vi "move.vi"(0 "value( disatance or angle)":dbl=1000.0 format="%#_13g", 1 "Speed precent":dbl(slide)=1.0 scale=0.0..1.0, 2 "mode":string="S") -> ()   [LabVIEW 2017]
uses:
  <vilib>/myRIO/Express VI/Onboard IO/PWM/PWM Express VI.xnode
  <vilib>/myRIO/Instrument Drivers/Onboard IO/PWM/vis/Set Duty Cycle and Frequency.vi
  <vilib>/myRIO/Instrument Drivers/Onboard IO/PWM/PWM.lvlib
  <vilib>/myRIO/Instrument Drivers/Onboard IO/PWM/typedefs/PWM Configuration.ctl
  <vilib>/myRIO/Common/Instrument Driver Framework/myRIO v1.0/PWM/typedefs/PWM Channels Enum.ctl
  <vilib>/myRIO/Common/Instrument Driver Framework/Utilities/typedefs/Generic FPGA Reference.ctl
  <vilib>/myRIO/Common/Instrument Driver Framework/Utilities/typedefs/myRIO v1.0 Reference.ctl
  <vilib>/myRIO/Common/Instrument Driver Framework/Utilities/typedefs/Hardware Version Enum.ctl
  <vilib>/myRIO/Common/Instrument Driver Framework/Utilities/typedefs/myRIO Generic Hardware Reference.ctl
  <vilib>/myRIO/Instrument Drivers/Onboard IO/PWM/typedefs/PWM Reference.ctl
  <vilib>/myRIO/Instrument Drivers/Onboard IO/PWM/vis/myRIO PWM Open.xnode
  <vilib>/myRIO/Common/Instrument Driver Framework/Utilities/vis/Is FPGA Ref Available.vi
  <vilib>/myRIO/Common/Instrument Driver Framework/myRIO v1.0/PWM/vis/myRIO v1.1 Open PWM.vi
  <vilib>/userdefined/High Color/nirio_resource_hc.ctl
  <vilib>/myRIO/Express VI/Onboard IO/DO/DO Express VI.xnode
  <vilib>/myRIO/Instrument Drivers/Onboard IO/DIO/vis/Write.vi
  <vilib>/myRIO/Instrument Drivers/Onboard IO/DIO/DIO.lvlib
  <vilib>/myRIO/Common/Instrument Driver Framework/myRIO v1.0/DIO/typedefs/DIO Channels Enum.ctl
  <vilib>/myRIO/Common/Instrument Driver Framework/myRIO v1.0/DIO/typedefs/DIO Channels List.ctl
  <vilib>/myRIO/Instrument Drivers/Onboard IO/DIO/typedefs/DIO Reference.ctl
  <vilib>/myRIO/Instrument Drivers/Onboard IO/DIO/vis/myRIO DIO Open.xnode
  <vilib>/myRIO/Common/Instrument Driver Framework/myRIO v1.0/DIO/vis/myRIO v1.1 Open DIO.vi
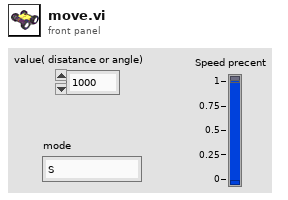
[diagram p1: front panel]
types:
  T1 = typedef "DIO.lvlib/DIO Reference.ctl" = cluster{"myRIO Reference":T2, "DIO Channels List":T6}
  T2 = typedef "myRIO Generic Hardware Reference.ctl" = cluster{"myRIO Model":T3, "myRIO Hardware Reference":T4}
  T3 = typedef "Hardware Version Enum.ctl" = enum16{"Unknown", "myRIO-1900", "myRIO-1950", "roboRIO", "NI ELVIS RIO CM"}
  T4 = typedef "myRIO v1.0 Reference.ctl" = cluster{"Generic FPGA Reference":T5, "Allow multiple opens":bool}
  T5 = typedef "Generic FPGA Reference.ctl" = refnum<k20>
  T6 = typedef "DIO Channels List.ctl" = T7[]
  T7 = typedef "DIO Channels Enum.ctl" = enum16{"Not Connected", "C/DIO0", "C/DIO1", "C/DIO2", "C/DIO3", "C/DIO4", "C/DIO5", "C/DIO6", "C/DIO7", "A/DIO0", "A/DIO1", "A/DIO2", "A/DIO3", "A/DIO4", "A/DIO5", "A/DIO6", "A/DIO7", "A/DIO8", "A/DIO9", "A/DIO10", "A/DIO11", "A/DIO12", "A/DIO13", "A/DIO14", "A/DIO15", "B/DIO0", "B/DIO1", "B/DIO2", "B/DIO3", "B/DIO4", "B/DIO5", "B/DIO6", "B/DIO7", "B/DIO8", "B/DIO9", "B/DIO10", "B/DIO11", "B/DIO12", "B/DIO13", "B/DIO14", "B/DIO15", "LED0", "LED1", "LED2", "LED3", "Button0", "DIO/DIO0", "DIO/DIO1", "DIO/DIO2", "DIO/DIO3", "DIO/DIO4", "DIO/DIO5", "DIO/DIO6", "DIO/DIO7", "DIO/DIO8", "DIO/DIO9", "SPI/CS0", "SPI/CS1", "SPI/CS2", "SPI/CS3", "LED RADIO (Green)", "LED RADIO (Red)", "LED COMM (Green)", "LED COMM (Red)", "LED MODE (Green)", "LED MODE (Red)"}
  T8 = typedef "nirio_resource_hc.ctl" = tag
  T9 = typedef "PWM.lvlib/PWM Reference.ctl" = cluster{"myRIO Reference":T2, "PWM Channels Enum":T10, "PWM Configuration":T11}
  T10 = typedef "PWM Channels Enum.ctl" = enum16{"Not Connected", "C/PWM0", "C/PWM1", "A/PWM0", "A/PWM1", "A/PWM2", "B/PWM0", "B/PWM1", "B/PWM2", "PWM/PWM0", "PWM/PWM1", "PWM/PWM2", "PWM/PWM3", "PWM/PWM4", "PWM/PWM5", "PWM/PWM6", "PWM/PWM7", "PWM/PWM8", "PWM/PWM9"}
  T11 = typedef "PWM.lvlib/PWM Configuration.ctl" = cluster{"Frequency":dbl, "Duty Cycle":dbl}
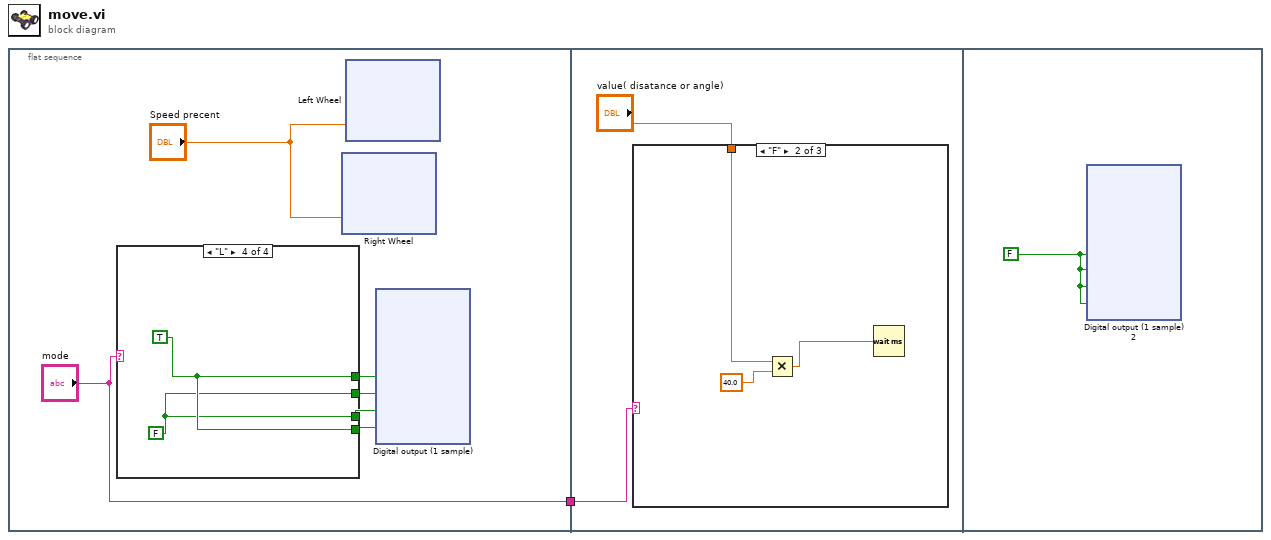
[diagram p0: block diagram]
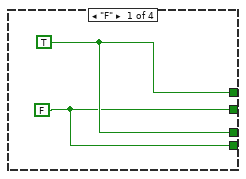
[diagram p2: hidden frame]
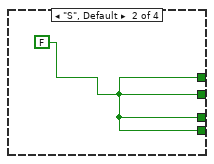
[diagram p3: hidden frame]
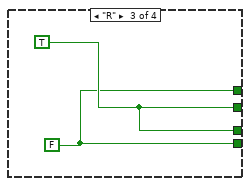
[diagram p4: hidden frame]
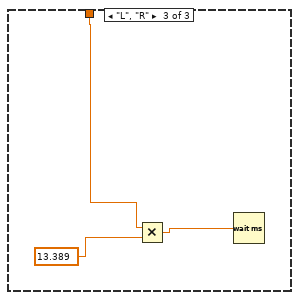
[diagram p6: hidden frame]
diagram:
  n1 = flat-sequence {
    tunnel: ["mode"] -> w1
    tunnel: w1 -> [w124]
    frame #0 {
      n2 = case shown="\"L\"" "mode" {
        tunnel: [w82 w83 w84 w87] -> w7
        tunnel: [w81 w83 w85 w86] -> w6
        tunnel: [w82 w83 w85 w86] -> w5
        tunnel: [w81 w83 w84 w87] -> w4
        frame "F" {
          w82 = TRUE
          w81 = FALSE
        }
        frame "S", Default {
          w83 = FALSE
        }
        frame "R" {
          w84 = FALSE
          w85 = TRUE
        }
        frame "L" {
          w86 = FALSE
          w87 = TRUE
        }
      }
      n3 = xnode "Right Wheel"("Duty Cycle"="Speed precent") -> ()  [unwired: 1 in, 1 out]
      n4 = xnode "Left Wheel"("Duty Cycle"="Speed precent") -> ()  [unwired: 1 in, 1 out]
      n5 = xnode "Digital output (1 sample)"("B/DIO0 (Pin 11)"=w7, "B/DIO1 (Pin 13)"=w6, "B/DIO2 (Pin 15)"=w5, "B/DIO3 (Pin 17)"=w4) -> ()  [unwired: 1 in, 1 out]
    }
    frame #1 {
      n6 = case shown="\"F\"" w124 {
        tunnel: "value( disatance or angle)" -> [_ w126 w128]
        frame Default {
        }
        frame "F" {
          n7 = Multiply(x=w126, y=40.0) -> (x*y=w127:dbl)
          n8 = Wait (ms)(milliseconds to wait=w127) -> ()  [unwired: 1 out]
        }
        frame "L", "R" {
          n9 = Multiply(x=w128, y=13.389) -> (x*y=w130:dbl)
          n10 = Wait (ms)(milliseconds to wait=w130) -> ()  [unwired: 1 out]
        }
      }
    }
    frame #2 {
      w131 = FALSE ("B/DIO0 (Pin 11)")
      n11 = xnode "Digital output (1 sample) 2"("B/DIO0 (Pin 11)"=w131, "B/DIO1 (Pin 13)"=w131, "B/DIO2 (Pin 15)"=w131, "B/DIO3 (Pin 17)"=w131) -> ()  [unwired: 1 in, 1 out]
    }
  }
